vi "Execute SQL Command.vi"(4 "error in":errorcluster, 6 "SQL Command":string, 7 "Connection In":refnum<k7>) -> (0 "error out":errorcluster, 1 "records effected":i32, 3 "Connection Out":refnum<k7>)   [LabVIEW 2020, in "ADO Database Drivers.lvlib"]
uses:
  ADO Database Drivers.lvlib
  <vilib>/Utility/error.llb/Error Cluster From Error Code.vi
  <vilib>/ErrorRing/Error Ring.xnode
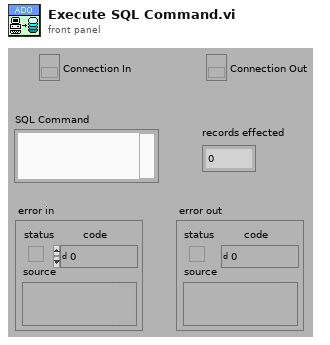
[diagram p1: front panel]
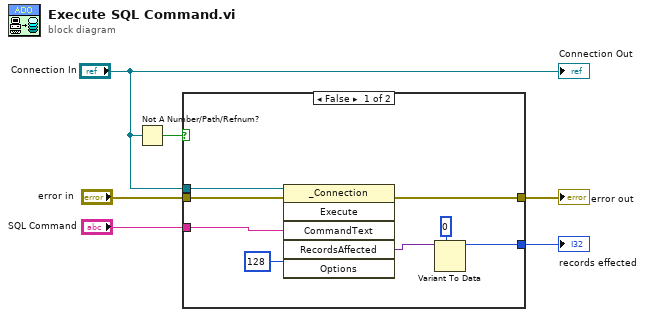
[diagram p0: block diagram]
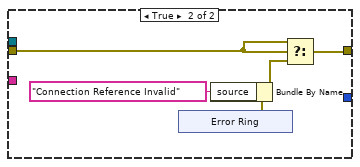
[diagram p2: hidden frame]
diagram:
  n1 = Not A Number/Path/Refnum?(number/path/refnum="Connection In") -> (NaN/Path/Refnum?=w2:bool)
  n2 = case shown="False" w2 {
    tunnel: [w12 _] -> w6
    tunnel: "SQL Command" -> [w11 _]
    tunnel: "error in" -> [w10 w17]
    tunnel: [w8 w16] -> w3
    tunnel: "Connection In" -> [w7 _]
    frame False {
      n3 = invoke class="_Connection" method="Execute"(reference=w7, error in=w10, "CommandText"=w11, "Options"=128) -> (error out=w8:errorcluster, "RecordsAffected"=w14:variant)  [unwired: 2 in, 4 out]
      n4 = Variant To Data(type=0, Variant=w14) -> (data=w12:i32)  [unwired: 1 in, 1 out]
    }
    frame True {
      n5 = xnode "Error Ring"() -> ("error out"=w19:errorcluster)
      n6 = Bundle By Name(cluster=w19, "source"="Connection Reference Invalid") -> (w15:errorcluster)
      n7 = Select(t=w17, s=w17, f=w15) -> (s? t:f=w16:errorcluster)
    }
  }
  "error out" <- w3
  "records effected" <- w6
  "Connection Out" <- "Connection In"
